vi "Time.Inline Delay.vi"(7 "Enable":bool=TRUE, 8 "error in (no error)":errorcluster, 9 "Wait(secs)":dbl, 10 "Wait(ms)":u32, 11 "error in top":errorcluster) -> (0 "error out":errorcluster, 3 "error out top":errorcluster)   [LabVIEW 2024, in "EQMF.lvlib" / "Time Utils.lvlib"]
uses:
  Time Utils.lvlib
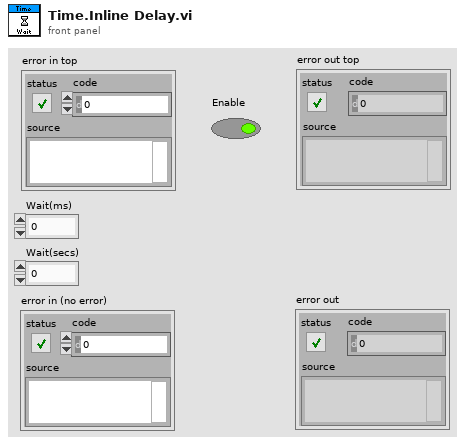
[diagram p1: front panel]
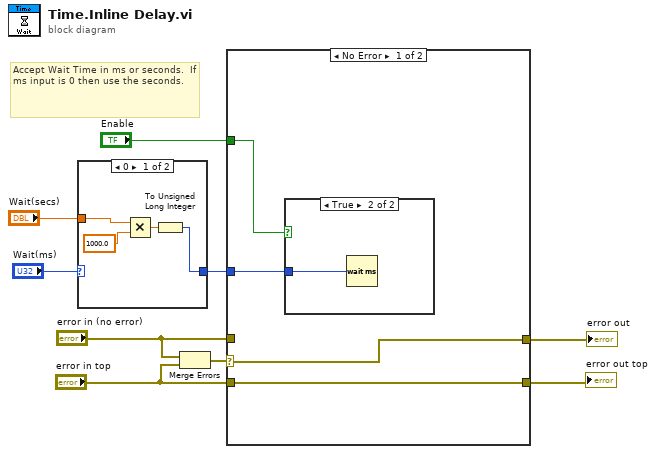
[diagram p0: block diagram]
diagram:
  # "Accept Wait Time in ms or seconds.  If ms input is 0 then use the seconds."
  n1 = case shown="0" "Wait(ms)" {
    selector: "Wait(ms)" -> [_ w14]
    tunnel: [w10 w14] -> w3
    tunnel: "Wait(secs)" -> [w13 _]
    frame 0 {
      n2 = Multiply(x=w13, y=1000.0) -> (x*y=w11:dbl)
      n3 = To Unsigned Long Integer(number=w11) -> (unsigned 32bit integer=w10:u32)
    }
    frame 1, Default {
    }
  }
  n4 = Merge Errors("error in (no error)", "error in top") -> (w7:errorcluster)
  n5 = case shown="No Error" w7 {
    selector: w7 -> [w17 _]
    tunnel: w3 -> [w18 _]
    tunnel: [w17 w20] -> w9
    tunnel: "error in top" -> [w16 w21]
    tunnel: [w16 w21] -> w8
    tunnel: "error in (no error)" -> [_ w20]
    tunnel: "Enable" -> [w15 _]
    frame No Error {
      n6 = case shown="True" w15 {
        tunnel: w18 -> [_ w19]
        frame False {
        }
        frame True {
          n7 = Wait (ms)(milliseconds to wait=w19) -> ()  [unwired: 1 out]
        }
      }
    }
    frame Error {
    }
  }
  "error out" <- w9
  "error out top" <- w8
